vi "Interpolation Filtering for Single Block.vi"() -> ()   [LabVIEW 2023]
doc: "Demonstrates how to use the DFD Nyquist Design VI to design an interpolation filter and use the DFD MRate Filtering for Single Block VI to process a single block of data with the interpolation filter.\n\nComplete the following steps to use this VI.\n1) Run the VI to filter the input signal with the default settings.\n2) Set <B>Zero Phase?</B> to True, run this VI again, and observe the Signals graph.\n3) Use the zoom tool to observe the samples at the beginning of the Interpolated Signal plot. \n4) Change the <B>Extension Type</B> option, run this VI again, and observe the plots.\n5) Examine the block diagram to learn how to set the specifications."
uses:
  <vilib>/addons/Digital Filter Design/_Objects.llb/DFD Multirate Filtering Mode.ctl
  <vilib>/addons/Digital Filter Design/Multirate.llb/DFD MRate Filtering for Single Block (Wfm).vi
  <vilib>/measure/NI_MABase.lvlib
  <vilib>/addons/Digital Filter Design/NI_DigFilterLicensed.lvlib
panel:
  in  "Extension Type":u16(ring) items=["Zero padding", "Symmetric", "Periodic"]
  out "Signals":waveform(dbl)[](graph)=[{"t0"=timestamp(0 s since 1904-01-01), "dt"=1.0, "Y"=[]}, {"t0"=timestamp(0 s since 1904-01-01), "dt"=1.0, "Y"=[]}]
  in  "Zero Phase?":bool=TRUE
  # "Select Help>>Show Context Help and move the cursor over the VI icon for more information."
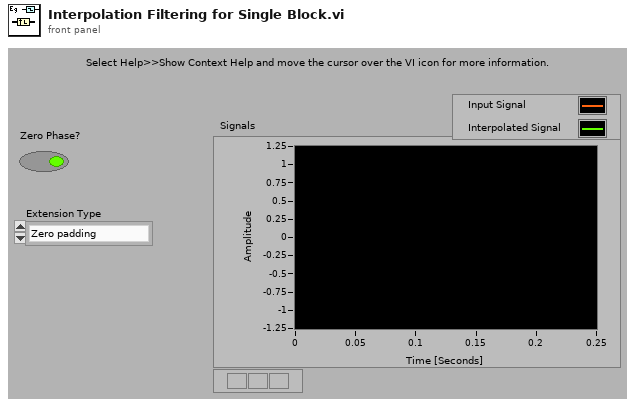
[diagram p1: front panel]
types:
  T1 = typedef "NI_DigFilterLicensed.lvlib/DFD Multirate Filtering Mode.ctl" = u16
  T2 = enum16{"Sine Wave", "Triangle Wave", "Square Wave", "Sawtooth Wave"}
  T3 = typedef "NI_DigFilterLicensed.lvlib/DFD Multirate Filter Obj.ctl" = cluster{"mMRate_Structure":enum16{"CIC", "FIR", "IIR", "Lattice"}, "mMRate_Mode":T4, "mMRate_Factor":i32, "mMRate_FIRParams":cluster{"mMRate_FIR_H":dbl[], "mMRate_FIR_IsNyquist?":bool, "mMRate_FIR_IsSymmetric?":bool}, "mMRate_CICParams":cluster{"mMRate_CIC_#Stage":i32, "mMRate_CIC_Lag":i32, "mMRate_CIC_Type":enum16{"Lowpass", "Highpass"}}, "mMRate_Order":i32, "mMRate_Version":string, "mMRate_Comments":string, "mMRate_RationalFactor":cluster{"mMRate_L":i32, "mMRate_M":i32}, "mMRate_Fs":dbl, "mMRate_Quantized?":bool, "mMRate_QFilterGain":dbl, "mMRate_CoefWl":i16, "mMRate_Scaling":cluster{"mMRate_ScaleByPowerOf2?":bool, "mMRate_ScaleType":T5}, "mMRate_InputWl":i16, "mMRate_OutputWl":i16, "mMRate_OutputMode":T6, "mMRate_MultMode":T7, "mMRate_BitPruning":bool, "mMRate_GainWl":i16, "mMRate_OutputFwl":i16, "mMRate_SumIwl":i16, "mMRate_InputIwl ":i16, "mMRate_SumWl":i16, "mMRate_CoefIwl":i16}
  T4 = typedef "NI_DigFilterLicensed.lvlib/DFD Multirate Mode.ctl" = i16
  T5 = typedef "NI_DigFilterLicensed.lvlib/DFD Coef Norm Type.ctl" = enum16{"No Norm", "Time Domain 1-Norm", "Time Domain 2-Norm", "Time Domain Inf-Norm"}
  T6 = typedef "NI_DigFilterLicensed.lvlib/DFD Round-off Mode.ctl" = enum16{"Nearest", "Truncation"}
  T7 = typedef "NI_DigFilterLicensed.lvlib/DFD FXP MRate Multiply Mode.ctl" = enum16{"Truncated", "Full"}
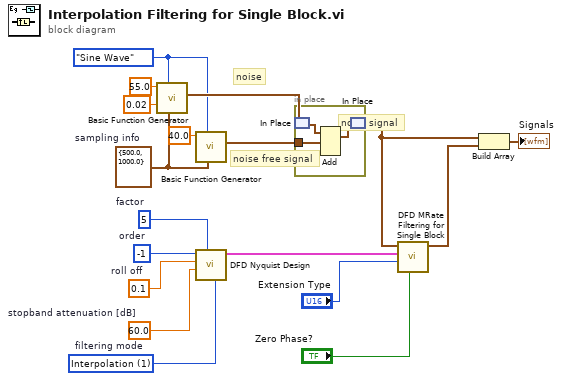
[diagram p0: block diagram]
diagram:
  w8 = 60.0  # stopband attenuation [dB]
  w9 = T1 1 items=["No Rate Change", "Interpolation", "Decimation"]  # filtering mode
  w10 = -1  # order
  w11 = 0.1  # roll off
  w3 = T2."Sine Wave" ("signal type")
  w17 = 5  # factor
  w13 = cluster{"Fs":dbl, "#s":dbl} {"Fs"=500.0, "#s"=1000.0}  # sampling info
  # "noisy signal"
  # "noise free signal"
  # "noise"
  n1 = call <vilib>:"Basic Function Generator.vi"("sampling info"=w13, "signal type"=w3, "amplitude"=0.02, "frequency"=55.0) -> ("signal out"=w14:waveform(dbl))  [unwired: 5 in, 2 out]
  n2 = call <vilib>:"Basic Function Generator.vi"("sampling info"=w13, "signal type"=w3, "frequency"=40.0) -> ("signal out"=w12:waveform(dbl))  [unwired: 6 in, 2 out]
  n3 = call <vilib>:"DFD Nyquist Design.vi"("filtering mode"=w9, "factor"=w17, "stopband attenuation [dB]"=w8, "roll off"=w11, "order"=w10) -> ("multirate filter out"=w7:T3)  [unwired: 3 in, 3 out]
  n4 = in-place {
    in-place-border: w12 -> [w20]
    n5 = in-place-match #1(w14) -> (w21:waveform(dbl))
    n6 = Add(1:w20, 2:w21) -> (0:w19:waveform(dbl))  [unwired: 1 in, 1 out]
    n7 = in-place-match #1(w19) -> (w4:waveform(dbl))
  }
  n8 = call-poly <vilib>:"DFD MRate Filtering for Single Block.vi"("zero phase? (T)"="Zero Phase?", "extension type"="Extension Type", "multirate filter"=w7, "signal in"=w4) -> ("signal out"=w1:waveform(dbl))  [unwired: 1 in, 6 out]
  n9 = Build Array(w4, w1) -> (→"Signals":waveform(dbl)[])
